vi "Query Motor Position (TRIAX).vi"(7 "Mono System # (0)":T1, 8 "error in (no error)":errorcluster, 11 "VISA resource name":refnum<visa-resource-name>) -> (0 "error out":errorcluster, 2 "wavelength":dbl[unit], 3 "VISA resource name out":refnum<visa-resource-name>)   [LabVIEW 2017, in "JY-SPEX-TRIAX.lvlib"]
doc: "Queries the current wavelength setting according to the base grating (1200 grooves/mm).\n\n<B>Note: only works with TRIAX series monochromators.</B>"
uses:
  JY-SPEX-TRIAX.lvlib
  controls.llb/Monochromator System Number.ctl
  Spectrometer Config.vi
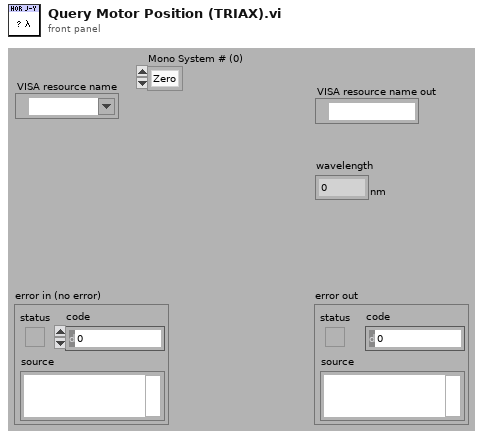
[diagram p1: front panel]
types:
  T1 = typedef "JY-SPEX-TRIAX.lvlib/Monochromator System Number.ctl" = enum16{"Zero", "One"}
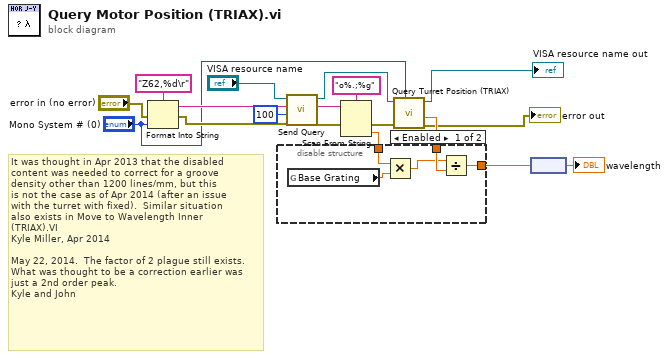
[diagram p0: block diagram]
diagram:
  # "It was thought in Apr 2013 that the disabled\ncontent was needed to correct for a groove\ndensity other than 1200 lines/mm, but this\nis not the case as of Apr 2014 (after an issue\nwith the turret with fixed).  Similar situation\nalso exists in Move to Wavelength Inner\n(TRIAX).VI\nKyle Miller, Apr 2014\n\nMay 22, 2014.  The factor of 2 plague still exists.\nWhat was thought to be a correction earlier was\njust a 2nd order peak.\nKyle and John"
  n1 = Format Into String(format string="Z62,%d\r", error in="error in (no error)", "Mono System # (0)") -> (resulting string=w11:string, error out=w9:errorcluster)  [unwired: 1 in]
  n2 = call "Send Query.vi"("error in (no error)"=w9, "byte count"=u32 100, "write buffer"=w11, "VISA resource name"="VISA resource name") -> ("error out"=w14:errorcluster, "read buffer"=w16:string, "VISA resource name out"=w8:refnum<visa-resource-name>)  [unwired: 5 out]
  n3 = Scan From String(format string="o%.;%g", input string=w16, error in=w14) -> (error out=w2:errorcluster, output 1=w7:dbl)  [unwired: 1 in, 3 out]
  n4 = call "Query Turret Position (TRIAX).vi"("Mono System # (0)"="Mono System # (0)", "error in (no error)"=w2, "VISA resource name"=w8) -> ("error out"=→"error out":errorcluster, "Groove Density"=w6:dbl[unit], "VISA resource name out"=→"VISA resource name out":refnum<visa-resource-name>)  [unwired: 4 in, 2 out]
  n5 = disable-structure shown="Enabled" {
    disable-tunnel: w7 -> [w23 w24]
    disable-tunnel: w6 -> [w21 _]
    disable-tunnel: [w19 w24] -> w5
    frame Enabled {
      n6 = global read "Spectrometer Config.vi" "Base Grating"() -> (w22:dbl[unit])
      n7 = Multiply(x=w23, y=w22) -> (x*y=w20:dbl[unit])
      n8 = Divide(x=w20, y=w21) -> (x/y=w19:dbl)
    }
    frame Disabled {
    }
  }
  n9 = node(w5) -> (→"wavelength":dbl[unit])
